vi "results to tag bus.vi"(9 "indices":T1, 10 "data cluster":T2, 11 "tag bus in":T3) -> (3 "tag bus out":T3)   [LabVIEW 2013, in "Temperature Controller Logic runtime.lvclass"]
uses:
  Temperature Controller Logic runtime.lvclass
  <vilib>/NI/Tag Bus/table/data table.ctl
  result user data.ctl
  configuration/result data indices.ctl
  <vilib>/NI/Tag Bus/table/data polymorphs/write one/write U8.vi
  <vilib>/NI/Tag Bus/table/data polymorphs/write one/write Double.vi
  <vilib>/NI/Tag Bus/table/data table.lvlib
  configuration/Temperature Controller Logic configuration.lvclass
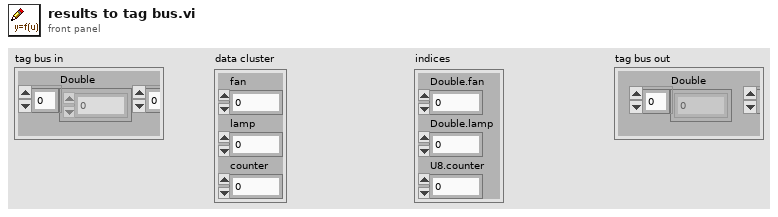
[diagram p1: front panel]
types:
  T1 = typedef "Temperature Controller Logic configuration.lvclass/result data indices.ctl" = cluster{"Double.fan":i32, "Double.lamp":i32, "U8.counter":i32}
  T2 = typedef "Temperature Controller Logic runtime.lvclass/result user data.ctl" = cluster{"fan":dbl, "lamp":dbl, "counter":u8}
  T3 = typedef "tag bus.lvlib/data table.lvlib/data table.ctl" = cluster{"Double":dbl[], "Single":sgl[], "I64":i64[], "I32":i32[], "I16":i16[], "I8":i8[], "U64":u64[], "U32":u32[], "U16":u16[], "U8":u8[], "Boolean":bool[], "String":string[], "Array of Double":cluster{"DBL Array":dbl[]}[], "Array of Single":cluster{"SGL Array":sgl[]}[], "Array of I64":cluster{"I64 Array":i64[]}[], "Array of I32":cluster{"I32 Array":i32[]}[], "Array of I16":cluster{"I16 Array":i16[]}[], "Array of I8":cluster{"I8 Array":i8[]}[], "Array of U64":cluster{"U64 Array":u64[]}[], "Array of U32":cluster{"U32 Array":u32[]}[], "Array of U16":cluster{"U16 Array":u16[]}[], "Array of U8":cluster{"U8 Array":u8[]}[], "Array of Boolean":cluster{"Boolean Array":bool[]}[], "Array of String":cluster{"String Array":string[]}[]}
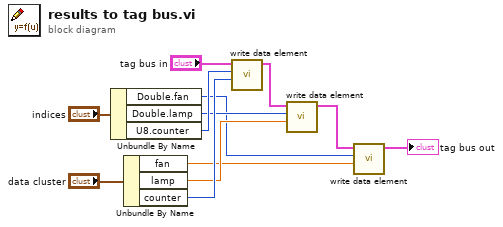
[diagram p0: block diagram]
diagram:
  n1 = Unbundle By Name("indices") -> ("Double.fan"=w4:i32, "Double.lamp"=w7:i32, "U8.counter"=w10:i32)
  n2 = Unbundle By Name("data cluster") -> ("fan"=w3:dbl, "lamp"=w6:dbl, "counter"=w9:u8)
  n3 = call-poly <vilib>:"write data element.vi"("value"=w9, "index"=w10, "data table in"="tag bus in") -> ("data table out"=w5:T3)  [unwired: 8 in]
  n4 = call-poly <vilib>:"write data element.vi"("value"=w6, "index"=w7, "data table in"=w5) -> ("data table out"=w2:T3)  [unwired: 8 in]
  n5 = call-poly <vilib>:"write data element.vi"("value"=w3, "index"=w4, "data table in"=w2) -> ("data table out"=→"tag bus out":T3)  [unwired: 8 in]
